vi "Diagnostic Test.vi"(8 "error in (no error)":errorcluster, 11 "CAP-USB-1 in":refnum<class "CAP-USB-1.lvclass">) -> (0 "error out":errorcluster, 3 "CAP-USB-1 out":refnum<class "CAP-USB-1.lvclass">)   [LabVIEW 2014, in "CAP-USB-1.lvlib" / "CAP-USB-1.lvclass"]
uses:
  CAP-USB-1.lvclass
  CAP-USB-1.lvclass/CAP-USB-1.ctl
  API/CAP-USB/CAP-USB.lvlib
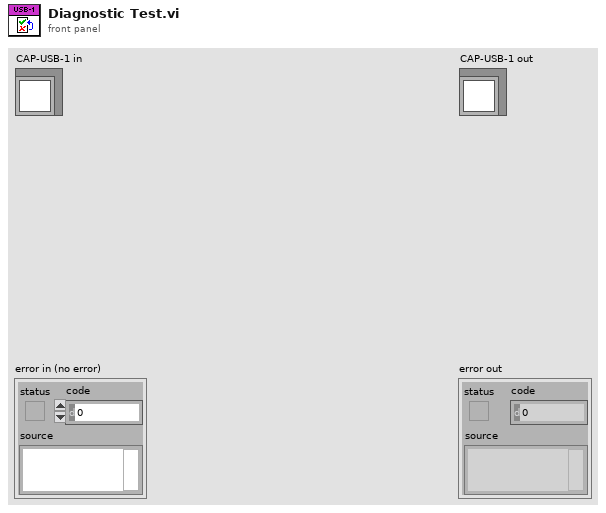
[diagram p1: front panel]
types:
  T1 = cluster{"Entradas":bool[], "Salidas":bool[], "Valor Encoder":u16, "Valor Transductores":u16[], "Orden Transd":u32[]}[]
  T2 = cluster{"Entradas":bool[], "Salidas":bool[], "Valor Encoder":u16, "Valor Transductores":u16[], "Orden Transd":u32[]}
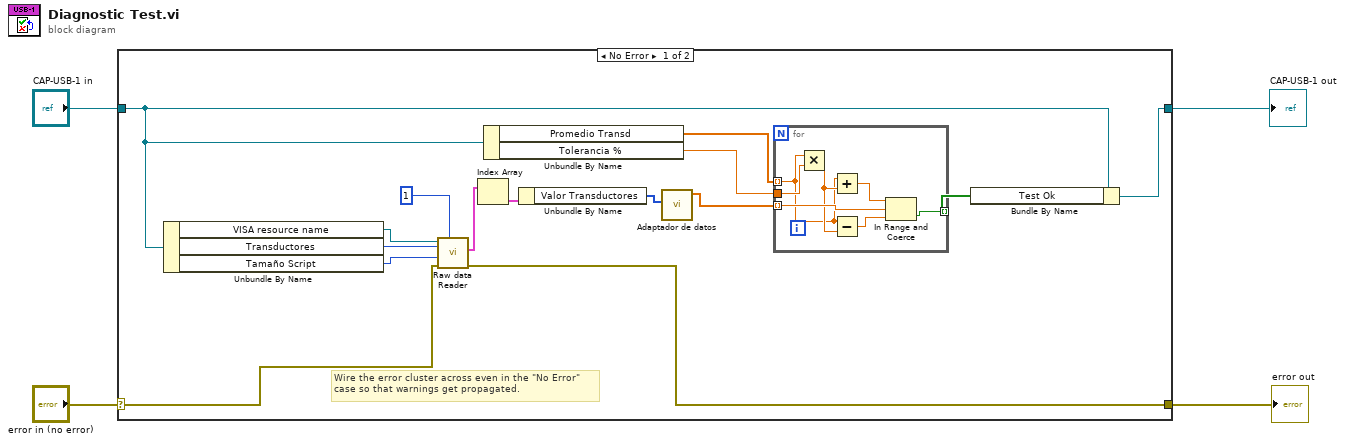
[diagram p0: block diagram]
diagram:
  n1 = case shown="No Error" "error in (no error)" {
    selector: "error in (no error)" -> [w16 w28]
    tunnel: [w15 w28] -> w3
    tunnel: [w6 w27] -> w1
    tunnel: "CAP-USB-1 in" -> [w8 w27]
    frame No Error {
      # "Wire the error cluster across even in the \"No Error\"\ncase so that warnings get propagated."
      n2 = Unbundle By Name(w8) -> ("VISA resource name"=w19:refnum<visa-resource-name>, "Transductores"=w18:u64, "Tamaño Script"=w17:i32)
      n3 = call "Raw data Reader.vi"("Num de tramas"=1, "error in (no error)"=w16, "Tamaño Script"=w17, "TRANSDUCTORES"=w18, "VISA Refnum in"=w19) -> ("error out"=w15:errorcluster, "Raw data"=w13:T1)  [unwired: 2 in, 1 out]
      n4 = Index Array(array=w13) -> (element=w12:T2)  [unwired: 1 in]
      n5 = Unbundle By Name(w8) -> ("Promedio Transd"=w11:sgl[], "Tolerancia %"=w5:sgl)
      n6 = Unbundle By Name(w12) -> ("Valor Transductores"=w10:u16[])
      n7 = call "Adaptador de datos.vi"("Transductores"=w10) -> ("Transductores"=w9:sgl[])  [unwired: 8 in, 2 out]
      n8 = for {
        tunnel: w11 -> [w21] mode=indexing
        tunnel: w5 -> [w25]
        tunnel: w9 -> [w26] mode=indexing
        tunnel: [w20] -> w7 mode=indexing
        n9 = Multiply(x=w21, y=w25) -> (x*y=w22:sgl)
        n10 = Add(x=w21, y=w22) -> (x+y=w24:sgl)
        n11 = Subtract(x=w21, y=w22) -> (x-y=w23:sgl)
        n12 = In Range and Coerce(upper limit=w24, x=w26, lower limit=w23) -> (In Range?=w20:bool)  [unwired: 1 out]
      }
      n13 = Bundle By Name(cluster=w8, "Test Ok"=w7) -> (w6:refnum<class "CAP-USB-1.lvclass">)
    }
    frame Error {
    }
  }
  "error out" <- w3
  "CAP-USB-1 out" <- w1
